vi "HiPAP sim.vi"(8 "Sample period HiPAP (ms)":dbl, 10 "Eta in":dbl[](array[numeric]), 11 "HiPAP std":dbl) -> (1 "Eta out":dbl[](array[numeric]))   [LabVIEW 2014]
uses:
  <vilib>/Analysis/NI_AALBase.lvlib
panel:
  out "x >= y?":bool
  out "x+y 2":dbl
  out "abs(x)":dbl[](array[numeric])
  out "element":dbl
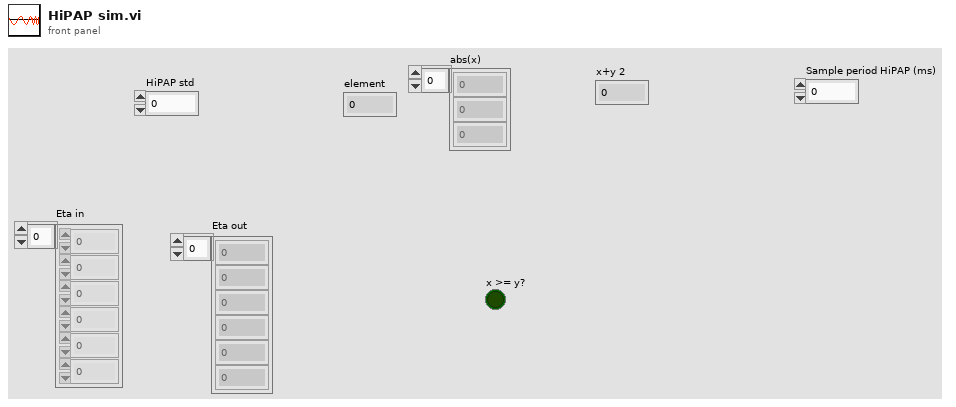
[diagram p1: front panel]
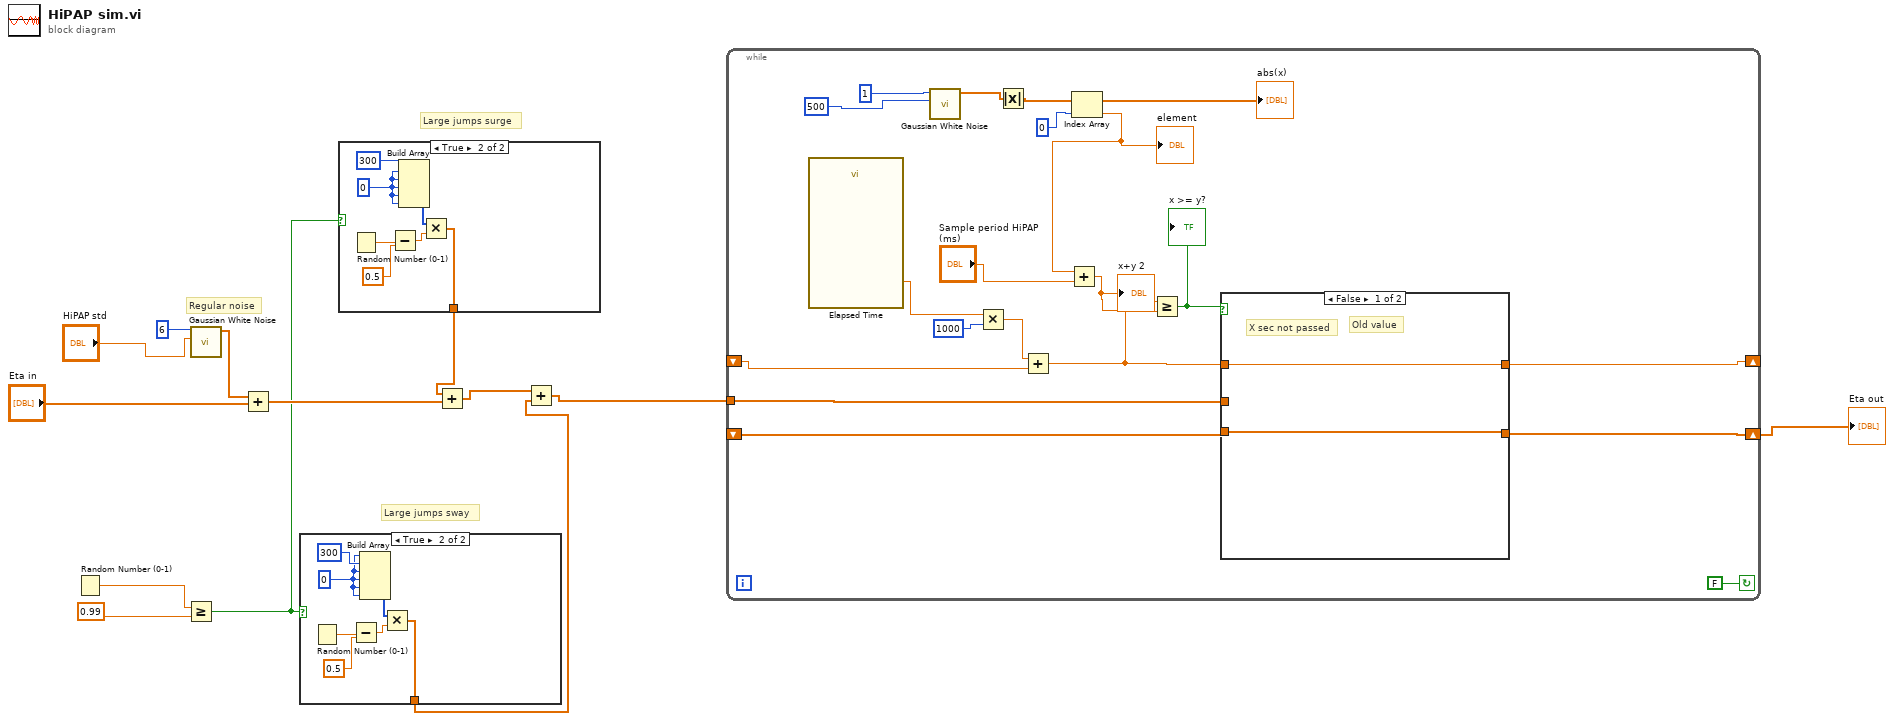
[diagram p0: block diagram]
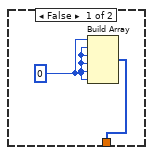
[diagram p2: hidden frame]
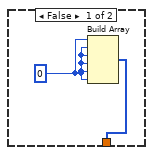
[diagram p3: hidden frame]
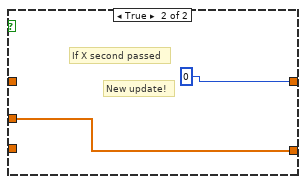
[diagram p4: hidden frame]
diagram:
  # "Large jumps sway"
  # "Large jumps surge"
  # "Regular noise"
  n1 = Random Number (0-1)() -> (number: 0 to 1=w6:dbl)
  n2 = Greater Or Equal?(x=w6, y=0.99) -> (x >= y?=w1:bool)
  n3 = call <vilib>:"Gaussian White Noise.vi"("standard deviation"="HiPAP std", "samples"=6) -> ("Gaussian noise pattern"=w12:dbl[])  [unwired: 8 in, 1 out]
  n4 = Add(x=w12, y="Eta in") -> (x+y=w11:dbl[])
  n5 = case shown="True" w1 {
    tunnel: [w15 w22] -> w5
    frame False {
      w14 = 0
      n6 = Build Array(w14, w14, w14, w14, w14, w14) -> (w15:i32[])
    }
    frame True {
      w16 = 0
      n7 = Random Number (0-1)() -> (number: 0 to 1=w20:dbl)
      n8 = Subtract(x=w20, y=0.5) -> (x-y=w19:dbl)
      n9 = Build Array(w16, 300, w16, w16, w16, w16) -> (w21:i32[])
      n10 = Multiply(x=w21, y=w19) -> (x*y=w22:dbl[])
    }
  }
  n11 = case shown="True" w1 {
    tunnel: [w24 w31] -> w10
    frame False {
      w23 = 0
      n12 = Build Array(w23, w23, w23, w23, w23, w23) -> (w24:i32[])
    }
    frame True {
      w25 = 0
      n13 = Random Number (0-1)() -> (number: 0 to 1=w29:dbl)
      n14 = Subtract(x=w29, y=0.5) -> (x-y=w28:dbl)
      n15 = Build Array(300, w25, w25, w25, w25, w25) -> (w30:i32[])
      n16 = Multiply(x=w30, y=w28) -> (x*y=w31:dbl[])
    }
  }
  n17 = Add(x=w10, y=w11) -> (x+y=w4:dbl[])
  n18 = Add(x=w4, y=w5) -> (x+y=w3:dbl[])
  n19 = while {
    tunnel: w3 -> [w34]
    shift-right: [w49] -> w9
    shift-left: _ -> [w33]
    shift-right: [w48] -> _
    shift-left: _ -> [w47]
    stop <- FALSE continue-if-true
    n20 = call "Elapsed Time"() -> ("Elapsed Time (s)"=w37:dbl)  [unwired: 12 in, 7 out]
    n21 = call <vilib>:"Gaussian White Noise.vi"("standard deviation"=500, "samples"=1) -> ("Gaussian noise pattern"=w43:dbl[])  [unwired: 8 in, 1 out]
    n22 = Multiply(x=w37, y=1000) -> (x*y=w35:dbl)
    n23 = Absolute Value(x=w43) -> (abs(x)=w41:dbl[])
    "abs(x)" <- w41
    n24 = Add(x=w35, y=w47) -> (x+y=w46:dbl)
    n25 = Index Array(array=w41, index=0) -> (element=w39:dbl)
    "element" <- w39
    n26 = Add(x=w39, y="Sample period HiPAP (ms)") -> (x+y=w42:dbl)
    "x+y 2" <- w42
    n27 = Greater Or Equal?(x=w46, y=w42) -> (x >= y?=w38:bool)
    "x >= y?" <- w38
    n28 = case shown="False" w38 {
      tunnel: w33 -> [w52 _]
      tunnel: [w52 w53] -> w49
      tunnel: w34 -> [_ w53]
      tunnel: w46 -> [w51 _]
      tunnel: [w51 0] -> w48
      frame False {
        # "Old value"
        # "X sec not passed"
      }
      frame True {
        # "New update!"
        # "If X second passed"
      }
    }
  }
  "Eta out" <- w9
